vi "Write Command.vi"(8 "error in (no error)":errorcluster, 10 "Command Data":T1, 11 "F4T in":refnum<class "F4T.lvclass">) -> (0 "error out":errorcluster, 3 "F4T out":refnum<class "F4T.lvclass">)   [LabVIEW 2018, in "F4T.lvlib" / "F4T.lvclass"]
doc: "Write Command for Watlow F4T."
uses:
  F4T.lvclass
  Custom Controls/Command Data.ctl
  F4T.lvclass/F4T.ctl
  C:/Program Files/National Instruments/LabVIEW 2018/instr.lib/Watlow Std Bus/Public/Watbus.dll
  Program Files/National Instruments/LabVIEW 2018/instr.lib/Watlow Std Bus/Public/Watbus.dll
  PPLs/Temp Chamber/Parent/Temp Chamber.lvlibp/Temp Chamber.lvclass
  C:/Projects/LabVIEW/PPLs/Temp Chamber/Parent/Temp Chamber.lvlibp/Temp Chamber.lvclass
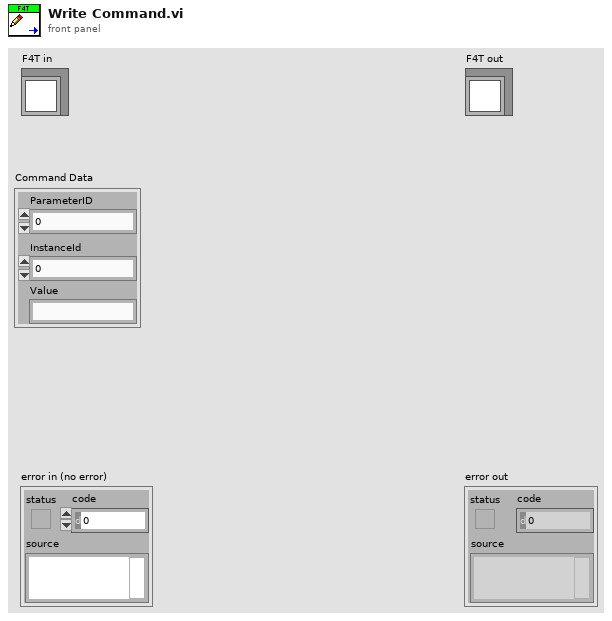
[diagram p1: front panel]
types:
  T1 = typedef "F4T.lvlib/F4T.lvclass/Command Data.ctl" = cluster{"ParameterID":u32, "InstanceId":u32, "Value":string}
  T2 = typedef "Temp Chamber.lvlibp/Temp Chamber.lvclass/Temp Units.ctl" = enum16{"Celsius", "Fahrenheit", "Kelvin", "Rankine"}
  T3 = typedef "F4T.lvlib/F4T.lvclass/Control Data.ctl" = cluster{"DeviceType ":u32, "Zone":u32}
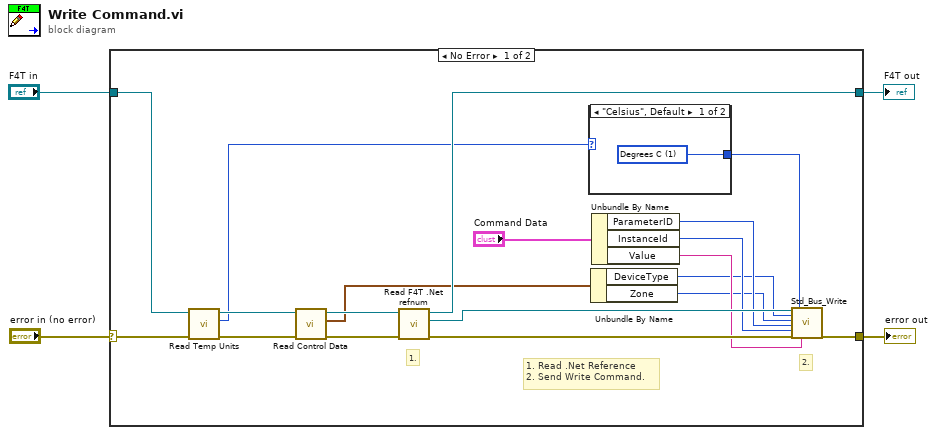
[diagram p0: block diagram]
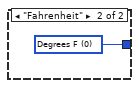
[diagram p2: hidden frame]
diagram:
  n1 = case shown="No Error" "error in (no error)" {
    selector: "error in (no error)" -> [w8 w27]
    tunnel: [w17 w27] -> w3
    tunnel: [w16 w26] -> w1
    tunnel: "F4T in" -> [w9 w26]
    frame No Error {
      # "1. Read .Net Reference\n2. Send Write Command."
      # "2."
      # "1."
      n2 = call "Read Temp Units.vi"("error in (no error)"=w8, "Temp Chamber in"=w9) -> ("error out"=w6:errorcluster, "Temp Units"=w5:T2, "Temp Chamber out"=w7:refnum<class "F4T.lvclass">)  [unwired: 7 in]
      n3 = call "Read Control Data.vi"("error in (no error)"=w6, "F4T in"=w7) -> ("error out"=w15:errorcluster, "Control Data"=w13:T3, "F4T out"=w14:refnum<class "F4T.lvclass">)  [unwired: 7 in]
      n4 = call "Read F4T .Net refnum.vi"("error in (no error)"=w15, "F4T in"=w14) -> ("error out"=w23:errorcluster, "F4T .Net refnum"=w21:refnum<k24>, "F4T out"=w16:refnum<class "F4T.lvclass">)  [unwired: 7 in]
      n5 = case shown="\"Celsius\", Default" w5 {
        tunnel: [w24 w25] -> w10
        frame "Celsius", Default {
          w24 = u8 1 items=["Degrees F", "Degrees C"] ("TemperatureUnits")
        }
        frame "Fahrenheit" {
          w25 = u8 0 items=["Degrees F", "Degrees C"] ("TemperatureUnits")
        }
      }
      n6 = Unbundle By Name(w13) -> ("DeviceType"=w12:u32, "Zone"=w11:u32)
      n7 = Unbundle By Name("Command Data") -> ("ParameterID"=w20:u32, "InstanceId"=w19:u32, "Value"=w18:string)
      n8 = call <instrlib>:"Std_Bus_Write.vi"("ILabVIEW In"=w21, "deviceType"=w12, "Zone"=w11, "ParameterID"=w20, "InstanceId"=w19, "error in (no error)"=w23, "TemperatureUnits"=w10, "WriteValue"=w18) -> ("error out"=w17:errorcluster)  [unwired: 10 in, 1 out]
    }
    frame Error {
    }
  }
  "error out" <- w3
  "F4T out" <- w1
